vi "smooth timetraces.vi"(1 "smooth":bool, 7 "PMT data":i16[](array[numeric])=[0, 0, 0, 0], 9 "window size":i32, 11 "max window size":i32, 12 "sums in":T1) -> (8 "smoothed data":i32[](array[numeric]), 14 "sums out":T1)   [LabVIEW 2009]
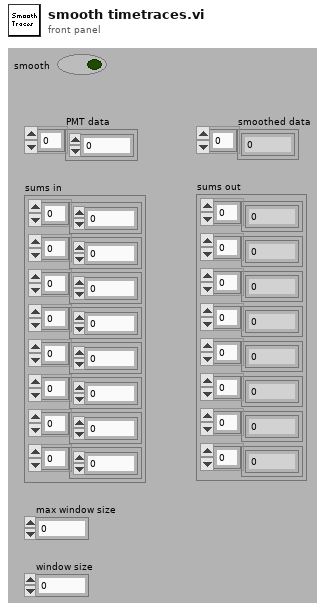
[diagram p1: front panel]
types:
  T1 = cluster{i16[], i16[], i16[], i16[], i16[], i16[], i16[], i16[]}
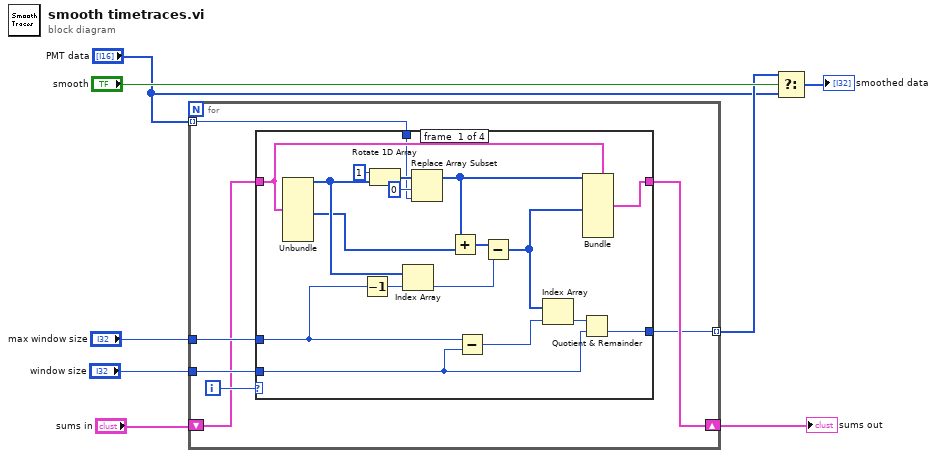
[diagram p0: block diagram]
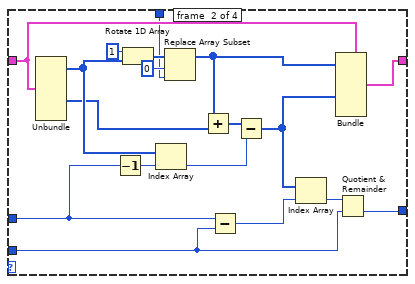
[diagram p2: hidden frame]
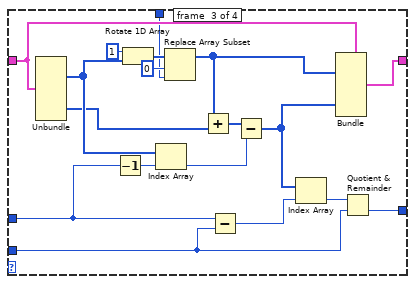
[diagram p3: hidden frame]
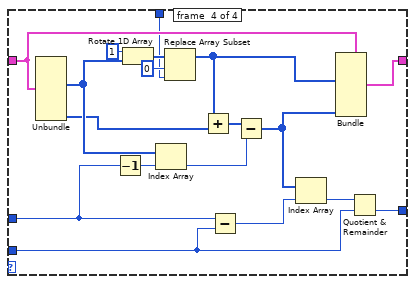
[diagram p4: hidden frame]
diagram:
  n1 = for {
    tunnel: "max window size" -> [w14]
    tunnel: [w13] -> w3 mode=indexing
    tunnel: "window size" -> [w12]
    tunnel: "PMT data" -> [w10] mode=indexing
    shift-right: [w15] -> w6
    shift-left: "sums in" -> [w9]
    i -> [w11]
    n2 = case shown="0, Default" w11 {
      tunnel: [w21 w43 w61 w79] -> w15
      tunnel: w9 -> [w23 w44 w62 w80]
      tunnel: w14 -> [w19 w37 w55 w73]
      tunnel: [w16 w34 w52 w70] -> w13
      tunnel: w12 -> [w17 w35 w53 w71]
      tunnel: w10 -> [w20 w38 w56 w74]
      frame #0 {
        n3 = Unbundle(w23) -> (w26:i16[], w25:i16[])  [unwired: 6 out]
        n4 = Decrement(x=w19) -> (x-1=w30:i32)
        n5 = Rotate 1D Array(1:w26, 2:1 ("n")) -> (0:w32:i16[])
        n6 = Index Array(array=w26, index=w30) -> (element=w29:i16)
        n7 = Replace Array Subset(array=w32, new element=w20, index=0 ("n")) -> (w24:i16[])
        n8 = Add(x=w24, y=w25) -> (x+y=w28:i16[])
        n9 = Subtract(x=w19, y=w17) -> (x-y=w27:i32)
        n10 = Subtract(x=w28, y=w29) -> (x-y=w22:i16[])
        n11 = Index Array(array=w22, index=w27) -> (element=w18:i16)
        n12 = Quotient & Remainder(x=w18, y=w17) -> (floor(x/y)=w16:i32)  [unwired: 1 out]
        n13 = Bundle(cluster=w23, w24, w22) -> (w21:T1)  [unwired: 6 in]
      }
      frame #1 {
        n14 = Unbundle(w44) -> (w42:i16[], w41:i16[])  [unwired: 6 out]
        n15 = Decrement(x=w37) -> (x-1=w48:i32)
        n16 = Rotate 1D Array(1:w42, 2:1 ("n")) -> (0:w50:i16[])
        n17 = Index Array(array=w42, index=w48) -> (element=w47:i16)
        n18 = Replace Array Subset(array=w50, new element=w38, index=0 ("n")) -> (w39:i16[])
        n19 = Add(x=w39, y=w41) -> (x+y=w46:i16[])
        n20 = Subtract(x=w37, y=w35) -> (x-y=w45:i32)
        n21 = Subtract(x=w46, y=w47) -> (x-y=w40:i16[])
        n22 = Index Array(array=w40, index=w45) -> (element=w36:i16)
        n23 = Bundle(cluster=w44, w39, w40) -> (w43:T1)  [unwired: 6 in]
        n24 = Quotient & Remainder(x=w36, y=w35) -> (floor(x/y)=w34:i32)  [unwired: 1 out]
      }
      frame #2 {
        n25 = Unbundle(w62) -> (w60:i16[], w59:i16[])  [unwired: 6 out]
        n26 = Decrement(x=w55) -> (x-1=w66:i32)
        n27 = Rotate 1D Array(1:w60, 2:1 ("n")) -> (0:w68:i16[])
        n28 = Index Array(array=w60, index=w66) -> (element=w65:i16)
        n29 = Replace Array Subset(array=w68, new element=w56, index=0 ("n")) -> (w57:i16[])
        n30 = Add(x=w57, y=w59) -> (x+y=w64:i16[])
        n31 = Subtract(x=w55, y=w53) -> (x-y=w63:i32)
        n32 = Subtract(x=w64, y=w65) -> (x-y=w58:i16[])
        n33 = Index Array(array=w58, index=w63) -> (element=w54:i16)
        n34 = Bundle(cluster=w62, w57, w58) -> (w61:T1)  [unwired: 6 in]
        n35 = Quotient & Remainder(x=w54, y=w53) -> (floor(x/y)=w52:i32)  [unwired: 1 out]
      }
      frame #3 {
        n36 = Unbundle(w80) -> (w78:i16[], w77:i16[])  [unwired: 6 out]
        n37 = Decrement(x=w73) -> (x-1=w84:i32)
        n38 = Rotate 1D Array(1:w78, 2:1 ("n")) -> (0:w86:i16[])
        n39 = Index Array(array=w78, index=w84) -> (element=w83:i16)
        n40 = Replace Array Subset(array=w86, new element=w74, index=0 ("n")) -> (w75:i16[])
        n41 = Add(x=w75, y=w77) -> (x+y=w82:i16[])
        n42 = Subtract(x=w73, y=w71) -> (x-y=w81:i32)
        n43 = Subtract(x=w82, y=w83) -> (x-y=w76:i16[])
        n44 = Index Array(array=w76, index=w81) -> (element=w72:i16)
        n45 = Bundle(cluster=w80, w75, w76) -> (w79:T1)  [unwired: 6 in]
        n46 = Quotient & Remainder(x=w72, y=w71) -> (floor(x/y)=w70:i32)  [unwired: 1 out]
      }
    }
  }
  "sums out" <- w6
  n47 = Select(t=w3, s="smooth", f="PMT data") -> (s? t:f=→"smoothed data":i32[])
